vi "Destroy All Dictionaries.vi"(8 "error in (no error)":errorcluster, 11 "DAQ":refnum<class "DAQ.lvclass">) -> (0 "error out":errorcluster, 3 "DAQ":refnum<class "DAQ.lvclass">)   [LabVIEW 2017, in "DAQ.lvclass"]
doc: "Developed by Kevin Thompson\nkevin@thompsonengineering.net\n\nCopyright 2018-2020\nThompson Engineering, LLC"
uses:
  DAQ.lvclass
  DAQ.lvclass/DAQ.ctl
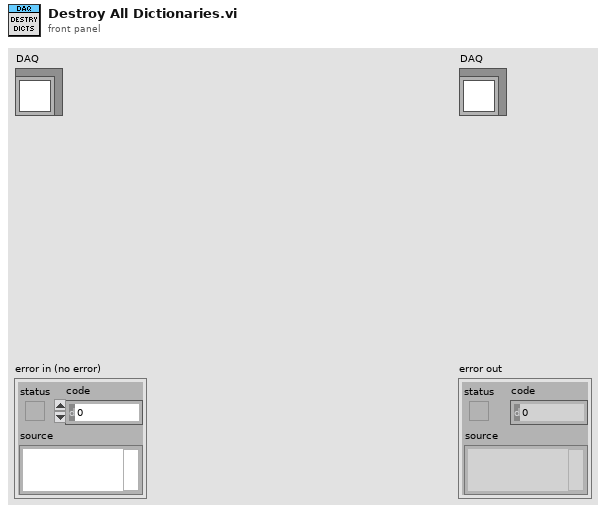
[diagram p1: front panel]
types:
  T1 = typedef "TD Dynamic CVT DVR--ref.ctl" = refnum<data-value>
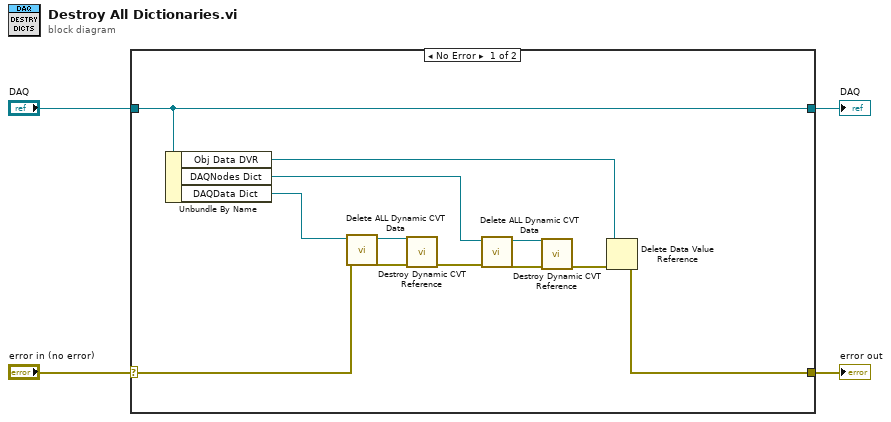
[diagram p0: block diagram]
diagram:
  n1 = case shown="No Error" "error in (no error)" {
    selector: "error in (no error)" -> [w9 w18]
    tunnel: [w5 w18] -> w3
    tunnel: [w16 w17] -> w1
    tunnel: "DAQ" -> [w16 w17]
    frame No Error {
      n2 = Unbundle By Name(w16) -> ("Obj Data DVR"=w7:refnum<data-value>, "DAQNodes Dict"=w8:T1, "DAQData Dict"=w14:T1)
      n3 = call <vilib>:"Delete ALL Dynamic CVT Data.vi"("error in (no error)"=w9, "dCVT DVR"=w14) -> ("error out"=w15:errorcluster, "dCVT DVR out"=w13:T1)  [unwired: 8 in]
      n4 = call <vilib>:"Destroy Dynamic CVT Reference.vi"("error in (no error)"=w15, "dCVT DVR"=w13) -> ("error out"=w10:errorcluster)  [unwired: 8 in, 1 out]
      n5 = call <vilib>:"Delete ALL Dynamic CVT Data.vi"("error in (no error)"=w10, "dCVT DVR"=w8) -> ("error out"=w11:errorcluster, "dCVT DVR out"=w12:T1)  [unwired: 8 in]
      n6 = call <vilib>:"Destroy Dynamic CVT Reference.vi"("error in (no error)"=w11, "dCVT DVR"=w12) -> ("error out"=w6:errorcluster)  [unwired: 8 in, 1 out]
      n7 = Delete Data Value Reference(data value reference=w7, error in=w6) -> (error out=w5:errorcluster)  [unwired: 1 out]
    }
    frame Error {
    }
  }
  "error out" <- w3
  "DAQ" <- w1
